vi "Un-load.vi"(8 "error in (no error)":errorcluster, 11 "Scope(Not Paths)":T1) -> (0 "error out":errorcluster)   [LabVIEW 2019, in "ClassLoader.lvlib"]
doc: "Unload cached data from memory according to the given scope."
uses:
  ClassLoader.lvlib
  Sub/Cache/Cache_Path Global.vi
  Sub/Cache/Cache_Hierarchy Global.vi
  Sub/Cache/Cache_Members Global.vi
  <vilib>/Utility/Data Type/Member VI Info.ctl
  Sub/Ctl/Ctl_Member Map.ctl
  Sub/Cache/Cache_PPL Global.vi
  Sub/Ctl/Ctl_PPL Details.ctl
  Sub/Cache/Cache_Info Global.vi
  Sub/Ctl/Ctl_Class Info.ctl
  Sub/Ctl/Ctl_Un-load Scope.ctl
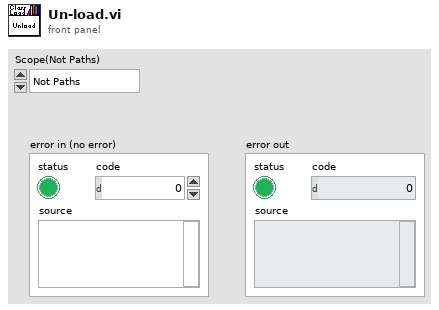
[diagram p1: front panel]
types:
  T1 = typedef "ClassLoader.lvlib/Ctl_Un-load Scope.ctl" = enum16{"Not Paths", "Not Paths nor Hierarchies", "All"}
  T2 = typedef "ClassLoader.lvlib/Ctl_Class Info.ctl" = cluster{"Name":string, "Qualified Name":string, "Internal Path":string}
  T3 = typedef "ClassLoader.lvlib/Ctl_Member Map.ctl" = map{string, T4}
  T4 = typedef "Member VI Info.ctl" = cluster{"qualified name":string, "path":path, "access scope":enum32{"invalid scope", "public", "private", "protected", "community"}, "is dynamic dispatch":bool}
  T5 = typedef "ClassLoader.lvlib/Ctl_PPL Details.ctl" = cluster{"Name":string, "Path":path, "Version":string}
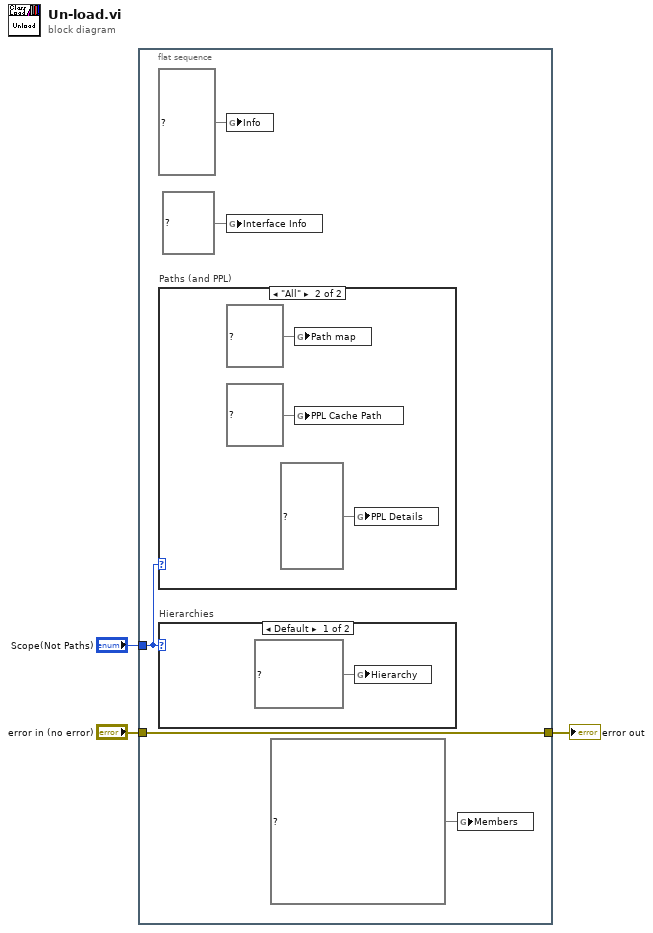
[diagram p0: block diagram]
diagram:
  n1 = flat-sequence {
    tunnel: "error in (no error)" -> [w8]
    tunnel: [w8] -> w2
    tunnel: "Scope(Not Paths)" -> [w7]
    frame #0 {
      n2 = case "Paths (and PPL)" shown="\"All\"" w7 {
        frame Default {
        }
        frame "All" {
          n3 = global write "Cache_Path Global.vi" "Path map"(map{string, path} {} ("Path map")) -> ()
          n4 = global write "Cache_PPL Global.vi" "PPL Cache Path"(map{string, path} {} ("PPL Cache Path")) -> ()
          n5 = global write "Cache_PPL Global.vi" "PPL Details"(map{string, T5} {} ("PPL Details")) -> ()
        }
      }
      n6 = case "Hierarchies" shown="Default" w7 {
        frame Default {
          n7 = global write "Cache_Hierarchy Global.vi" "Hierarchy"(map{string, string[]} {} ("Hierarchy")) -> ()
        }
        frame "Not Paths nor Hierarchies" {
        }
      }
      n8 = global write "Cache_Info Global.vi" "Info"(map{string, T2} {} ("Info")) -> ()
      n9 = global write "Cache_Info Global.vi" "Interface Info"(map{string, bool} {} ("Interface Info")) -> ()
      n10 = global write "Cache_Members Global.vi" "Members"(map{string, T3} {} ("Members")) -> ()
    }
  }
  "error out" <- w2
